vi "Reef Align Play Path Field Position.vi"(1 "PID Constants swerve":T1={"P Gain"=0.09, "I Gain"=0.0, "D Gain"=0.0, "F Gain"=0.08, "I Zone"=0.0, "Min Output"=-1.0, "Max Output"=1.0}, 2 "Operation":T2=enum."Reef Align", 3 "Auto Data":T14={"Auto Velocities"=[{"X Velocity"=-1.8462498434907955, "Y Velocity"=7.056933814139086, "Rotational \nVelocity"=-0.0}, {"X Velocity"=-1.991747061129249, "Y Velocity"=7.535671418858484, "Rotational \nVelocity"=-7.2}, {"X Velocity"=-2.1476402119148625, "Y Velocity"=8.011584634482254, "Rotational \nVelocity"=-10.052643775939941}, {"X Velocity"=-2.306896278662117, "Y Velocity"=8.486490625788083, "Rotational \nVelocity"=-10.052643775939941}, {"X Velocity"=-2.4695100913190724, "Y Velocity"=8.960371657345226, "Rotational \nVelocity"=-10.052643775939941}, {"X Velocity"=-2.635476396794092, "Y Velocity"=9.433210017677535, "Rotational \nVelocity"=-10.052643775939941}, {"X Velocity"=-2.6685615639393947, "Y Velocity"=9.423903981638178, "Rotational \nVelocity"=-10.052643775939941}, {"X Velocity"=-2.701613872254829, "Y Velocity"=9.414481906133277, "Rotational \nVelocity"=-10.052643775939941}, {"X Velocity"=-2.7346329147570203, "Y Velocity"=9.404943907179781, "Rotational \nVelocity"=-10.052643775939941}, {"X Velocity"=-2.6263332099505634, "Y Velocity"=8.91566678376851, "Rotational \nVelocity"=-10.052643775939941}, {"X Velocity"=-2.5146351435076726, "Y Velocity"=8.427271425386172, "Rotational \nVelocity"=-10.052643775939941}, {"X Velocity"=-2.3995435908884546, "Y Velocity"=7.939775651158667, "Rotational \nVelocity"=-10.052643775939941}, {"X Velocity"=-2.2810635107418573, "Y Velocity"=7.453197256780454, "Rotational \nVelocity"=-10.052643775939941}, {"X Velocity"=-2.1591999448009993, "Y Velocity"=6.967554014150215, "Rotational \nVelocity"=-10.052643775939941}, {"X Velocity"=-2.0339580177769934, "Y Velocity"=6.482863671006963, "Rotational \nVelocity"=-10.052643775939941}, {"X Velocity"=-1.9053429372511914, "Y Velocity"=5.99914395056661, "Rotational \nVelocity"=-10.052643775939941}, {"X Velocity"=-1.7733599935659488, "Y Velocity"=5.516412551158996, "Rotational \nVelocity"=-10.052643775939941}, {"X Velocity"=-1.63801455971383, "Y Velocity"=5.034687145865371, "Rotational \nVelocity"=-10.052643775939941}, {"X Velocity"=-1.4993120912253046, "Y Velocity"=4.553985382156366, "Rotational \nVelocity"=-10.052643775939941}, {"X Velocity"=-1.3572581260549188, "Y Velocity"=4.074324881530425, "Rotational \nVelocity"=-10.052643775939941}, {"X Velocity"=-1.2118582844659433, "Y Velocity"=3.595723239152738, "Rotational \nVelocity"=-10.052643775939941}, {"X Velocity"=-1.0631182689134988, "Y Velocity"=3.118198023494648, "Rotational \nVelocity"=-10.052643775939941}, {"X Velocity"=-0.9110438639261721, "Y Velocity"=2.641766775973572, "Rotational \nVelocity"=-10.052643775939941}, {"X Velocity"=-0.7556409359861169, "Y Velocity"=2.166447010593411, "Rotational \nVelocity"=-10.052643775939941}, {"X Velocity"=-0.5969154334076338, "Y Velocity"=1.692256213585474, "Rotational \nVelocity"=-10.052643775939941}, {"X Velocity"=-0.4348733862142511, "Y Velocity"=1.2192118430499221, "Rotational \nVelocity"=-10.052643775939941}, {"X Velocity"=-0.26947258503234844, "Y Velocity"=0.7473487535270189, "Rotational \nVelocity"=-9.867414283752396}, {"X Velocity"=-0.1001328097589842, "Y Velocity"=0.2768976473427397, "Rotational \nVelocity"=-2.6674142837523886}, {"X Velocity"=-0.0, "Y Velocity"=0.0, "Rotational \nVelocity"=-0.0}], "Auto Positions"=[{"x"=0.8100058273974486, "y"=-3.967975741983552, "th"=5.222202301025391}, {"x"=0.7603878706355013, "y"=-3.830783760791278, "th"=5.0782023010253905}, {"x"=0.7073688364180365, "y"=-3.68418791485404, "th"=4.877149425506592}, {"x"=0.6509487247450543, "y"=-3.5281882041718386, "th"=4.676096549987793}, {"x"=0.5911275356165546, "y"=-3.3627846287446737, "th"=4.475043674468994}, {"x"=0.5279052690325376, "y"=-3.1879771885725448, "th"=4.273990798950195}, {"x"=0.46128192499300325, "y"=-3.0037658836554524, "th"=4.072937923431397}, {"x"=0.39465858095346884, "y"=-2.8195545787383596, "th"=3.8718850479125977}, {"x"=0.32803523691393444, "y"=-2.6353432738212668, "th"=3.6708321723937987}, {"x"=0.26141189287440003, "y"=-2.451131968904174, "th"=3.469779296875}, {"x"=0.198189626290383, "y"=-2.276324528732045, "th"=3.2687264213562015}, {"x"=0.1383684371618834, "y"=-2.1109209533048796, "th"=3.0676735458374025}, {"x"=0.0819483254889012, "y"=-1.954921242622678, "th"=2.8666206703186035}, {"x"=0.02892929127143639, "y"=-1.8083253966854402, "th"=2.6655677947998044}, {"x"=-0.020688665490511016, "y"=-1.671133415493166, "th"=2.4645149192810054}, {"x"=-0.06690554479694102, "y"=-1.5433452990458556, "th"=2.2634620437622064}, {"x"=-0.10972134664785363, "y"=-1.4249610473435088, "th"=2.0624091682434074}, {"x"=-0.14913607104324883, "y"=-1.315980660386126, "th"=1.8613562927246083}, {"x"=-0.18514971798312663, "y"=-1.2164041381737067, "th"=1.6603034172058093}, {"x"=-0.21776228746748705, "y"=-1.1262314807062512, "th"=1.4592505416870103}, {"x"=-0.24697377949633004, "y"=-1.0454626879837594, "th"=1.2581976661682113}, {"x"=-0.27278419406965565, "y"=-0.9740977600062313, "th"=1.0571447906494127}, {"x"=-0.29519353118746383, "y"=-0.9121366967736668, "th"=0.8560919151306141}, {"x"=-0.31420179084975464, "y"=-0.8595794982860661, "th"=0.6550390396118155}, {"x"=-0.329808973056528, "y"=-0.816426164543429, "th"=0.45398616409301695}, {"x"=-0.342015077807784, "y"=-0.7826766955457557, "th"=0.2529332885742184}, {"x"=-0.35082010510352263, "y"=-0.7583310912930461, "th"=0.055585002899170455}, {"x"=-0.3562240549437438, "y"=-0.7433893517853002, "th"=0.002236717224122664}, {"x"=-0.35822692732844763, "y"=-0.737851477022518, "th"=0.002236717224122664}], "Auto Commands"=[], "Zero Velocity?"=[]}, 4 "Motors":T3={"Drive Motors (NEO)"={"Left Front"={"DeviceStatus"={"status"=FALSE, "code"=0, "source"=""}, "Type"=enum."CAN", "PWM"={"PWM Channel"=enum."Invalid", "DeadBand"={"Name"="", "maxPositivePwm"=0, "minPositivePwm"=0, "centerPwm"=0, "maxNegativePwm"=0, "minNegativePwm"=0, "angularRange"=0}}, "CAN"={"Device Number"=1, "SetOutput VI Ref"=variant(refnum<vi> refnum), "GetOutput VI Ref"=variant(refnum<vi> refnum), "Enable VI Ref"=variant(refnum<vi> refnum), "Disable VI Ref"=variant(refnum<vi> refnum), "Data"=variant(cluster{"Ext ID":u32, "CAN Timeout":u32, "Inverted No WPILib":bool, "Has Configured Limit Sw":bool, "Has Configured Alt Encoder":bool, "SPARK Model":enum16{"SPARK MAX", "SPARK Flex", "Unknown"}, "CAN Max Retries":u32, "CAN Timeout (ms)":u32, "Status 0 Period (ms)":u32, "Status 1 Period (ms)":u32, "Status 2 Period (ms)":u32, "Status 3 Period (ms)":u32, "Status 4 Period (ms)":u32, "Status 5 Period (ms)":u32, "Status 6 Period (ms)":u32, "Status 7 Period (ms)":u32, "Status Frame Timeout (ms)":u32} {"Ext ID"=33882113, "CAN Timeout"=0, "Inverted No WPILib"=FALSE, "Has Configured Limit Sw"=FALSE, "Has Configured Alt Encoder"=FALSE, "SPARK Model"=enum."SPARK Flex", "CAN Max Retries"=5, "CAN Timeout (ms)"=20, "Status 0 Period (ms)"=10, "Status 1 Period (ms)"=250, "Status 2 Period (ms)"=20, "Status 3 Period (ms)"=20, "Status 4 Period (ms)"=20, "Status 5 Period (ms)"=20, "Status 6 Period (ms)"=20, "Status 7 Period (ms)"=20, "Status Frame Timeout (ms)"=500})}, "Invert"=FALSE, "DIO PWM"={"PWM \"Enable\" Channel"=enum."Invalid", "DIOChannel"=enum."Invalid", "PWM Rate"=0.0}}, "Left Back"={"DeviceStatus"={"status"=FALSE, "code"=0, "source"=""}, "Type"=enum."CAN", "PWM"={"PWM Channel"=enum."Invalid", "DeadBand"={"Name"="", "maxPositivePwm"=0, "minPositivePwm"=0, "centerPwm"=0, "maxNegativePwm"=0, "minNegativePwm"=0, "angularRange"=0}}, "CAN"={"Device Number"=3, "SetOutput VI Ref"=variant(refnum<vi> refnum), "GetOutput VI Ref"=variant(refnum<vi> refnum), "Enable VI Ref"=variant(refnum<vi> refnum), "Disable VI Ref"=variant(refnum<vi> refnum), "Data"=variant(cluster{"Ext ID":u32, "CAN Timeout":u32, "Inverted No WPILib":bool, "Has Configured Limit Sw":bool, "Has Configured Alt Encoder":bool, "SPARK Model":enum16{"SPARK MAX", "SPARK Flex", "Unknown"}, "CAN Max Retries":u32, "CAN Timeout (ms)":u32, "Status 0 Period (ms)":u32, "Status 1 Period (ms)":u32, "Status 2 Period (ms)":u32, "Status 3 Period (ms)":u32, "Status 4 Period (ms)":u32, "Status 5 Period (ms)":u32, "Status 6 Period (ms)":u32, "Status 7 Period (ms)":u32, "Status Frame Timeout (ms)":u32} {"Ext ID"=33882115, "CAN Timeout"=0, "Inverted No WPILib"=FALSE, "Has Configured Limit Sw"=FALSE, "Has Configured Alt Encoder"=FALSE, "SPARK Model"=enum."SPARK Flex", "CAN Max Retries"=5, "CAN Timeout (ms)"=20, "Status 0 Period (ms)"=10, "Status 1 Period (ms)"=250, "Status 2 Period (ms)"=20, "Status 3 Period (ms)"=20, "Status 4 Period (ms)"=20, "Status 5 Period (ms)"=20, "Status 6 Period (ms)"=20, "Status 7 Period (ms)"=20, "Status Frame Timeout (ms)"=500})}, "Invert"=FALSE, "DIO PWM"={"PWM \"Enable\" Channel"=enum."Invalid", "DIOChannel"=enum."Invalid", "PWM Rate"=0.0}}, "Right Front"={"DeviceStatus"={"status"=FALSE, "code"=0, "source"=""}, "Type"=enum."CAN", "PWM"={"PWM Channel"=enum."Invalid", "DeadBand"={"Name"="", "maxPositivePwm"=0, "minPositivePwm"=0, "centerPwm"=0, "maxNegativePwm"=0, "minNegativePwm"=0, "angularRange"=0}}, "CAN"={"Device Number"=5, "SetOutput VI Ref"=variant(refnum<vi> refnum), "GetOutput VI Ref"=variant(refnum<vi> refnum), "Enable VI Ref"=variant(refnum<vi> refnum), "Disable VI Ref"=variant(refnum<vi> refnum), "Data"=variant(cluster{"Ext ID":u32, "CAN Timeout":u32, "Inverted No WPILib":bool, "Has Configured Limit Sw":bool, "Has Configured Alt Encoder":bool, "SPARK Model":enum16{"SPARK MAX", "SPARK Flex", "Unknown"}, "CAN Max Retries":u32, "CAN Timeout (ms)":u32, "Status 0 Period (ms)":u32, "Status 1 Period (ms)":u32, "Status 2 Period (ms)":u32, "Status 3 Period (ms)":u32, "Status 4 Period (ms)":u32, "Status 5 Period (ms)":u32, "Status 6 Period (ms)":u32, "Status 7 Period (ms)":u32, "Status Frame Timeout (ms)":u32} {"Ext ID"=33882117, "CAN Timeout"=0, "Inverted No WPILib"=FALSE, "Has Configured Limit Sw"=FALSE, "Has Configured Alt Encoder"=FALSE, "SPARK Model"=enum."SPARK Flex", "CAN Max Retries"=5, "CAN Timeout (ms)"=20, "Status 0 Period (ms)"=10, "Status 1 Period (ms)"=250, "Status 2 Period (ms)"=20, "Status 3 Period (ms)"=20, "Status 4 Period (ms)"=20, "Status 5 Period (ms)"=20, "Status 6 Period (ms)"=20, "Status 7 Period (ms)"=20, "Status Frame Timeout (ms)"=500})}, "Invert"=FALSE, "DIO PWM"={"PWM \"Enable\" Channel"=enum."Invalid", "DIOChannel"=enum."Invalid", "PWM Rate"=0.0}}, "Right Back"={"DeviceStatus"={"status"=FALSE, "code"=0, "source"=""}, "Type"=enum."CAN", "PWM"={"PWM Channel"=enum."Invalid", "DeadBand"={"Name"="", "maxPositivePwm"=0, "minPositivePwm"=0, "centerPwm"=0, "maxNegativePwm"=0, "minNegativePwm"=0, "angularRange"=0}}, "CAN"={"Device Number"=7, "SetOutput VI Ref"=variant(refnum<vi> refnum), "GetOutput VI Ref"=variant(refnum<vi> refnum), "Enable VI Ref"=variant(refnum<vi> refnum), "Disable VI Ref"=variant(refnum<vi> refnum), "Data"=variant(cluster{"Ext ID":u32, "CAN Timeout":u32, "Inverted No WPILib":bool, "Has Configured Limit Sw":bool, "Has Configured Alt Encoder":bool, "SPARK Model":enum16{"SPARK MAX", "SPARK Flex", "Unknown"}, "CAN Max Retries":u32, "CAN Timeout (ms)":u32, "Status 0 Period (ms)":u32, "Status 1 Period (ms)":u32, "Status 2 Period (ms)":u32, "Status 3 Period (ms)":u32, "Status 4 Period (ms)":u32, "Status 5 Period (ms)":u32, "Status 6 Period (ms)":u32, "Status 7 Period (ms)":u32, "Status Frame Timeout (ms)":u32} {"Ext ID"=33882119, "CAN Timeout"=0, "Inverted No WPILib"=FALSE, "Has Configured Limit Sw"=FALSE, "Has Configured Alt Encoder"=FALSE, "SPARK Model"=enum."SPARK Flex", "CAN Max Retries"=5, "CAN Timeout (ms)"=20, "Status 0 Period (ms)"=10, "Status 1 Period (ms)"=250, "Status 2 Period (ms)"=20, "Status 3 Period (ms)"=20, "Status 4 Period (ms)"=20, "Status 5 Period (ms)"=20, "Status 6 Period (ms)"=20, "Status 7 Period (ms)"=20, "Status Frame Timeout (ms)"=500})}, "Invert"=FALSE, "DIO PWM"={"PWM \"Enable\" Channel"=enum."Invalid", "DIOChannel"=enum."Invalid", "PWM Rate"=0.0}}}, "Steer Motors (NEO)"={"Left Front"={"DeviceStatus"={"status"=FALSE, "code"=0, "source"=""}, "Type"=enum."CAN", "PWM"={"PWM Channel"=enum."Invalid", "DeadBand"={"Name"="", "maxPositivePwm"=0, "minPositivePwm"=0, "centerPwm"=0, "maxNegativePwm"=0, "minNegativePwm"=0, "angularRange"=0}}, "CAN"={"Device Number"=2, "SetOutput VI Ref"=variant(refnum<vi> refnum), "GetOutput VI Ref"=variant(refnum<vi> refnum), "Enable VI Ref"=variant(refnum<vi> refnum), "Disable VI Ref"=variant(refnum<vi> refnum), "Data"=variant(cluster{"Ext ID":u32, "CAN Timeout":u32, "Inverted No WPILib":bool, "Has Configured Limit Sw":bool, "Has Configured Alt Encoder":bool, "SPARK Model":enum16{"SPARK MAX", "SPARK Flex", "Unknown"}, "CAN Max Retries":u32, "CAN Timeout (ms)":u32, "Status 0 Period (ms)":u32, "Status 1 Period (ms)":u32, "Status 2 Period (ms)":u32, "Status 3 Period (ms)":u32, "Status 4 Period (ms)":u32, "Status 5 Period (ms)":u32, "Status 6 Period (ms)":u32, "Status 7 Period (ms)":u32, "Status Frame Timeout (ms)":u32} {"Ext ID"=33882114, "CAN Timeout"=0, "Inverted No WPILib"=TRUE, "Has Configured Limit Sw"=FALSE, "Has Configured Alt Encoder"=FALSE, "SPARK Model"=enum."SPARK MAX", "CAN Max Retries"=5, "CAN Timeout (ms)"=20, "Status 0 Period (ms)"=10, "Status 1 Period (ms)"=250, "Status 2 Period (ms)"=20, "Status 3 Period (ms)"=20, "Status 4 Period (ms)"=20, "Status 5 Period (ms)"=20, "Status 6 Period (ms)"=20, "Status 7 Period (ms)"=20, "Status Frame Timeout (ms)"=500})}, "Invert"=FALSE, "DIO PWM"={"PWM \"Enable\" Channel"=enum."Invalid", "DIOChannel"=enum."Invalid", "PWM Rate"=0.0}}, "Left Back"={"DeviceStatus"={"status"=FALSE, "code"=0, "source"=""}, "Type"=enum."CAN", "PWM"={"PWM Channel"=enum."Invalid", "DeadBand"={"Name"="", "maxPositivePwm"=0, "minPositivePwm"=0, "centerPwm"=0, "maxNegativePwm"=0, "minNegativePwm"=0, "angularRange"=0}}, "CAN"={"Device Number"=4, "SetOutput VI Ref"=variant(refnum<vi> refnum), "GetOutput VI Ref"=variant(refnum<vi> refnum), "Enable VI Ref"=variant(refnum<vi> refnum), "Disable VI Ref"=variant(refnum<vi> refnum), "Data"=variant(cluster{"Ext ID":u32, "CAN Timeout":u32, "Inverted No WPILib":bool, "Has Configured Limit Sw":bool, "Has Configured Alt Encoder":bool, "SPARK Model":enum16{"SPARK MAX", "SPARK Flex", "Unknown"}, "CAN Max Retries":u32, "CAN Timeout (ms)":u32, "Status 0 Period (ms)":u32, "Status 1 Period (ms)":u32, "Status 2 Period (ms)":u32, "Status 3 Period (ms)":u32, "Status 4 Period (ms)":u32, "Status 5 Period (ms)":u32, "Status 6 Period (ms)":u32, "Status 7 Period (ms)":u32, "Status Frame Timeout (ms)":u32} {"Ext ID"=33882116, "CAN Timeout"=0, "Inverted No WPILib"=TRUE, "Has Configured Limit Sw"=FALSE, "Has Configured Alt Encoder"=FALSE, "SPARK Model"=enum."SPARK MAX", "CAN Max Retries"=5, "CAN Timeout (ms)"=20, "Status 0 Period (ms)"=10, "Status 1 Period (ms)"=250, "Status 2 Period (ms)"=20, "Status 3 Period (ms)"=20, "Status 4 Period (ms)"=20, "Status 5 Period (ms)"=20, "Status 6 Period (ms)"=20, "Status 7 Period (ms)"=20, "Status Frame Timeout (ms)"=500})}, "Invert"=FALSE, "DIO PWM"={"PWM \"Enable\" Channel"=enum."Invalid", "DIOChannel"=enum."Invalid", "PWM Rate"=0.0}}, "Right Front"={"DeviceStatus"={"status"=FALSE, "code"=0, "source"=""}, "Type"=enum."CAN", "PWM"={"PWM Channel"=enum."Invalid", "DeadBand"={"Name"="", "maxPositivePwm"=0, "minPositivePwm"=0, "centerPwm"=0, "maxNegativePwm"=0, "minNegativePwm"=0, "angularRange"=0}}, "CAN"={"Device Number"=6, "SetOutput VI Ref"=variant(refnum<vi> refnum), "GetOutput VI Ref"=variant(refnum<vi> refnum), "Enable VI Ref"=variant(refnum<vi> refnum), "Disable VI Ref"=variant(refnum<vi> refnum), "Data"=variant(cluster{"Ext ID":u32, "CAN Timeout":u32, "Inverted No WPILib":bool, "Has Configured Limit Sw":bool, "Has Configured Alt Encoder":bool, "SPARK Model":enum16{"SPARK MAX", "SPARK Flex", "Unknown"}, "CAN Max Retries":u32, "CAN Timeout (ms)":u32, "Status 0 Period (ms)":u32, "Status 1 Period (ms)":u32, "Status 2 Period (ms)":u32, "Status 3 Period (ms)":u32, "Status 4 Period (ms)":u32, "Status 5 Period (ms)":u32, "Status 6 Period (ms)":u32, "Status 7 Period (ms)":u32, "Status Frame Timeout (ms)":u32} {"Ext ID"=33882118, "CAN Timeout"=0, "Inverted No WPILib"=TRUE, "Has Configured Limit Sw"=FALSE, "Has Configured Alt Encoder"=FALSE, "SPARK Model"=enum."SPARK MAX", "CAN Max Retries"=5, "CAN Timeout (ms)"=20, "Status 0 Period (ms)"=10, "Status 1 Period (ms)"=250, "Status 2 Period (ms)"=20, "Status 3 Period (ms)"=20, "Status 4 Period (ms)"=20, "Status 5 Period (ms)"=20, "Status 6 Period (ms)"=20, "Status 7 Period (ms)"=20, "Status Frame Timeout (ms)"=500})}, "Invert"=FALSE, "DIO PWM"={"PWM \"Enable\" Channel"=enum."Invalid", "DIOChannel"=enum."Invalid", "PWM Rate"=0.0}}, "Right Back"={"DeviceStatus"={"status"=FALSE, "code"=0, "source"=""}, "Type"=enum."CAN", "PWM"={"PWM Channel"=enum."Invalid", "DeadBand"={"Name"="", "maxPositivePwm"=0, "minPositivePwm"=0, "centerPwm"=0, "maxNegativePwm"=0, "minNegativePwm"=0, "angularRange"=0}}, "CAN"={"Device Number"=8, "SetOutput VI Ref"=variant(refnum<vi> refnum), "GetOutput VI Ref"=variant(refnum<vi> refnum), "Enable VI Ref"=variant(refnum<vi> refnum), "Disable VI Ref"=variant(refnum<vi> refnum), "Data"=variant(cluster{"Ext ID":u32, "CAN Timeout":u32, "Inverted No WPILib":bool, "Has Configured Limit Sw":bool, "Has Configured Alt Encoder":bool, "SPARK Model":enum16{"SPARK MAX", "SPARK Flex", "Unknown"}, "CAN Max Retries":u32, "CAN Timeout (ms)":u32, "Status 0 Period (ms)":u32, "Status 1 Period (ms)":u32, "Status 2 Period (ms)":u32, "Status 3 Period (ms)":u32, "Status 4 Period (ms)":u32, "Status 5 Period (ms)":u32, "Status 6 Period (ms)":u32, "Status 7 Period (ms)":u32, "Status Frame Timeout (ms)":u32} {"Ext ID"=33882120, "CAN Timeout"=0, "Inverted No WPILib"=TRUE, "Has Configured Limit Sw"=FALSE, "Has Configured Alt Encoder"=FALSE, "SPARK Model"=enum."SPARK MAX", "CAN Max Retries"=5, "CAN Timeout (ms)"=20, "Status 0 Period (ms)"=10, "Status 1 Period (ms)"=250, "Status 2 Period (ms)"=20, "Status 3 Period (ms)"=20, "Status 4 Period (ms)"=20, "Status 5 Period (ms)"=20, "Status 6 Period (ms)"=20, "Status 7 Period (ms)"=20, "Status Frame Timeout (ms)"=500})}, "Invert"=FALSE, "DIO PWM"={"PWM \"Enable\" Channel"=enum."Invalid", "DIOChannel"=enum."Invalid", "PWM Rate"=0.0}}}, "Pigeon2"={"DeviceStatus"={"status"=FALSE, "code"=0, "source"=""}, "Device Number"=21, "Type"=352321536, "Device ID"=352321557, "Handle"=22044056, "UsageFrame"=0, "Library Path"=path "libCTRE_PhoenixCCI.so"}, "Radii (ft)"={"Left Front Position"=[-0.9375, 0.9375], "Left Back Position"=[-0.9375, -0.9375], "Right Front Position"=[0.9375, 0.9375], "Right Back Position"=[0.9375, -0.9375]}} {"Radii (ft)"."Right Back Position" format="%.2f"; "Radii (ft)"."Right Front Position" format="%.2f"; "Radii (ft)"."Left Back Position" format="%.2f"; "Radii (ft)"."Left Front Position" format="%.2f"; "Pigeon2"."Type" items=["CAN"=352321536, "TalonSRX"=33554432]}) -> (0 "Align Good?":bool)   [LabVIEW 2023]
uses:
  swerve/Type Definitions/Data/Robot Velocities.ctl
  swerve/Type Definitions/Hardware/Swerve Drives/(NEO-NEO-ThroughBore-Pigeon2) Swerve.ctl
  swerve/Type Definitions/Hardware/4 Motor Sets/(NEO & NEO 550) 4 Motor Set.ctl
  <vilib>/Rock Robotics/WPI/MotorControl/WPI_MotorControlDeviceRef.ctl
  <vilib>/Rock Robotics/WPI/MotorControl/WPI_MotorControlType.ctl
  <vilib>/Rock Robotics/SystemInterfaces/DIO/FPGA_DIOPWMChannel.ctl
  <vilib>/Rock Robotics/WPI/PWM/WPI_PWMDeadband.ctl
  <vilib>/Rock Robotics/SystemInterfaces/DIO/FPGA_DIOChannel.ctl
  <vilib>/Rock Robotics/WPI/ThirdParty/Phoenix-LabVIEW/Pigeon IMU/CTRE_PigeonIMU_DeviceRef.ctl
  <vilib>/Rock Robotics/WPI/ThirdParty/Phoenix-LabVIEW/Pigeon IMU/CTRE_PigeonIMU_ConnectionType.ctl
  swerve/Type Definitions/Data/Pod Positions.ctl
  Implementation/Drive Operations.ctl
  <vilib>/Rock Robotics/WPI/ThirdParty/REV Robotics/REVLib/Typedef/Spark MAX Control Type.ctl
  <vilib>/Platform/TimedLoop/XDataNode/timing_clust.ctl
  <vilib>/Platform/TimedLoop/XDataNode/nitl_modes.ctl
  <vilib>/Platform/TimedLoop/XDataNode/wakeup.ctl
  <vilib>/Rock Robotics/WPI/DriverStation/WPI_DriverStationRobotMode2.ctl
  ba9e1e52-2e86-4a5f-ad71-bc975f8651a0.vi
  Framework/Robot Global Data.vi
  <vilib>/Platform/TimedLoop/XDataNode/XDataNode.xnode
  <vilib>/Platform/TimedLoop/XDataNode/XDNodeRunTimeDep.lvlib
panel:
  out "Delay":dbl=9.0
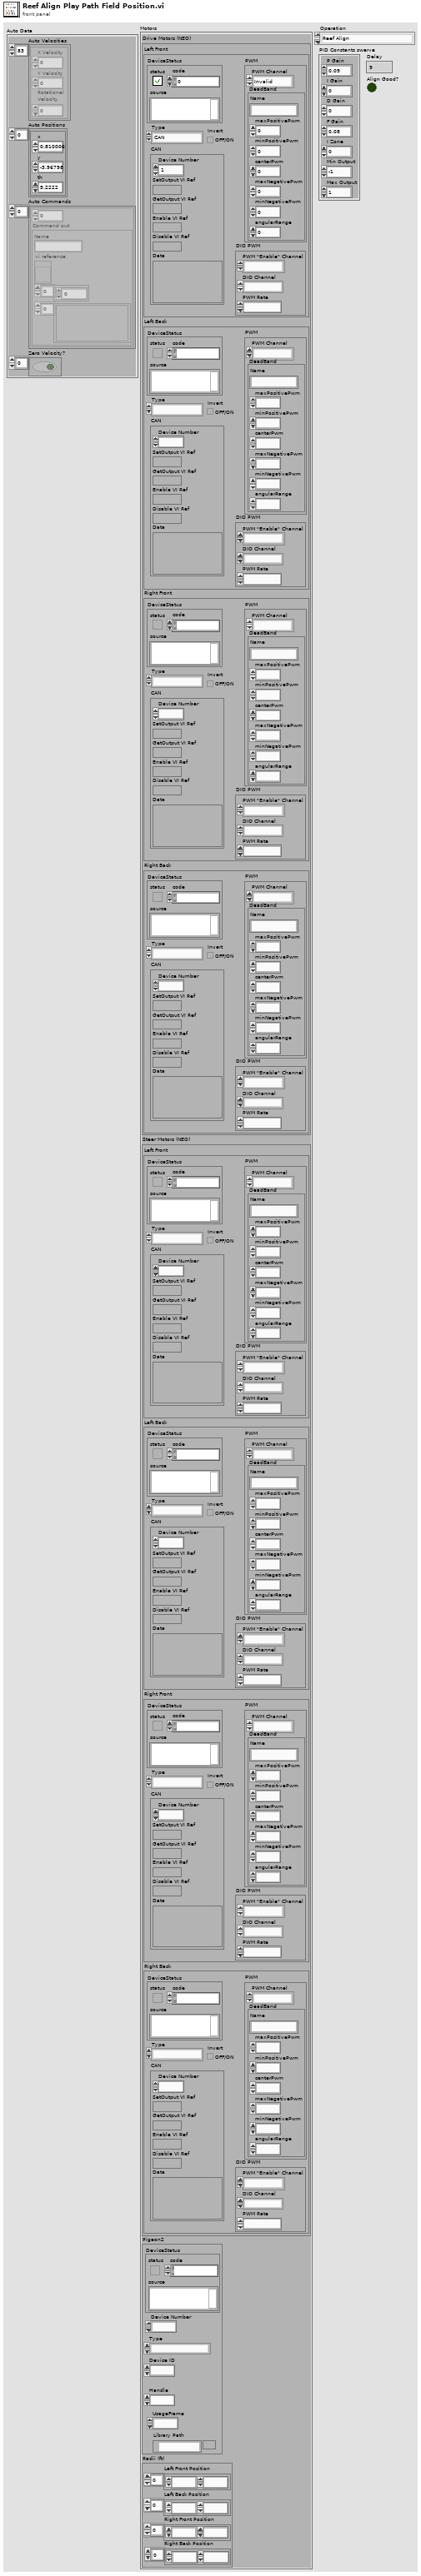
[diagram p1: front panel]
types:
  T1 = cluster{"P Gain":dbl, "I Gain":dbl, "D Gain":dbl, "F Gain":dbl, "I Zone":dbl, "Min Output":dbl, "Max Output":dbl}
  T2 = typedef "Drive Operations.ctl" = enum16{"Reserve", "Read Current", "Immediate", "Calibrate", "Reef Align", "Auto", "Old Reef Align"}
  T3 = typedef "(NEO-NEO-ThroughBore-Pigeon2) Swerve.ctl" = cluster{"Drive Motors (NEO)":T4, "Steer Motors (NEO)":T4, "Pigeon2":T10, "Radii (ft)":T12}
  T4 = typedef "(NEO & NEO 550) 4 Motor Set.ctl" = cluster{"Left Front":T5, "Left Back":T5, "Right Front":T5, "Right Back":T5}
  T5 = typedef "WPI_MotorControlDeviceRef.ctl" = cluster{"DeviceStatus":errorcluster, "Type":T6, "PWM":cluster{"PWM Channel":T7, "DeadBand":T8}, "CAN":cluster{"Device Number":u8, "SetOutput VI Ref":variant, "GetOutput VI Ref":variant, "Enable VI Ref":variant, "Disable VI Ref":variant, "Data":variant}, "Invert":bool, "DIO PWM":cluster{"PWM \"Enable\" Channel":T7, "DIOChannel":T9, "PWM Rate":dbl}}
  T6 = typedef "WPI_MotorControlType.ctl" = enum16{"PWM", "CAN", "DIO PWM"}
  T7 = typedef "FPGA_DIOPWMChannel.ctl" = enum8{"PWM 0", "PWM 1", "PWM 2", "PWM 3", "PWM 4", "PWM 5", "PWM 6", "PWM 7", "PWM 8", "PWM 9", "PWM MXP 0", "PWM MXP 1", "PWM MXP 2", "PWM MXP 3", "PWM MXP 4", "PWM MXP 5", "PWM MXP 6", "PWM MXP 7", "PWM MXP 8", "PWM MXP 9", "Invalid"}
  T8 = typedef "WPI_PWMDeadband.ctl" = cluster{"Name":string, "maxPositivePwm":i32, "minPositivePwm":i32, "centerPwm":i32, "maxNegativePwm":i32, "minNegativePwm":i32, "angularRange":u16}
  T9 = typedef "FPGA_DIOChannel.ctl" = enum8{"DIO 0", "DIO 1", "DIO 2", "DIO 3", "DIO 4", "DIO 5", "DIO 6", "DIO 7", "DIO 8", "DIO 9", "DIO MXP 0", "DIO MXP 1", "DIO MXP 2", "DIO MXP 3", "DIO MXP 4", "DIO MXP 5", "DIO MXP 6", "DIO MXP 7", "DIO MXP 8", "DIO MXP 9", "DIO MXP 10", "DIO MXP 11", "DIO MXP 12", "DIO MXP 13", "DIO MXP 14", "DIO MXP 15", "SPI Port CS1", "SPI Port CS2", "SPI Port CS3", "SPI Port MISO", "SPI Port MOSI", "Invalid"}
  T10 = typedef "CTRE_PigeonIMU_DeviceRef.ctl" = cluster{"DeviceStatus":errorcluster, "Device Number":u8, "Type":T11, "Device ID":u32, "Handle":u64, "UsageFrame":u32, "Library Path":path}
  T11 = typedef "CTRE_PigeonIMU_ConnectionType.ctl" = u32
  T12 = typedef "Pod Positions.ctl" = cluster{"Left Front Position":dbl[], "Left Back Position":dbl[], "Right Front Position":dbl[], "Right Back Position":dbl[]}
  T13 = typedef "Robot Velocities.ctl" = cluster{"X Velocity":dbl, "Y Velocity":dbl, "Rotational \nVelocity":dbl}
  T14 = cluster{"Auto Velocities":T13[], "Auto Positions":cluster{"x":dbl, "y":dbl, "th":dbl}[], "Auto Commands":cluster{dbl, "Command out":cluster{"Name":string, "vi reference":refnum<vi>, i32[], variant[]}}[], "Zero Velocity?":bool[]}
  T15 = typedef "Spark MAX Control Type.ctl" = enum16{"Percent VBus", "Voltage", "Velocity", "Position", "Smart Motion", "Current", "Smart Velocity", "MAXMotion Position", "MAXMotion Velocity"}
  T16 = cluster{"Left Front":dbl, "Left Back":dbl, "Right Front":dbl, "Right Back":dbl}
  T17 = cluster{"Time (s)":dbl, "Command out":cluster{"Name":string, "vi reference":refnum<vi>, i32[], variant[]}}
  T18 = cluster{dbl, "Command out":cluster{"Name":string, "vi reference":refnum<vi>, i32[], variant[]}}[]
  T19 = typedef "XDNodeRunTimeDep.lvlib/timing_clust.ctl" = cluster{"Expected End [f-1]":u64, "Actual End [f-1]":u64, "Finished Late? [f-1]":bool, "Expected End [i-1]":u64, "Actual End [i-1]":u64, "Finished Late? [i-1]":bool, "Expected Start [i]":u64, "Actual Start [i]":u64, "Expected Start [f]":u64, "Actual Start [f]":u64, "Source Name":string, "Structure Name":string, "Period":i64, "Deadline":i64, "Offset":i64, "Start":i64, "Priority":i32, "Timeout":i32, "Mode":T20, "Wakeup Reason":T21, "Error":errorcluster, "Source Type":string, "Secondary Source Type":string, "Global End Time":u64, "Global Start Time":u64, "Frame Duration":u64, "Iteration Duration":u64, "Assigned CPU":i32, "I/O Scan Engine Mode":u32}
  T20 = typedef "XDNodeRunTimeDep.lvlib/nitl_modes.ctl" = enum32{"No Change", "Process missed periods, maintain original phase", "Discard missed periods, maintain original phase", "Process missed periods, ignore original phase", "Discard missed periods, ignore original phase"}
  T21 = typedef "XDNodeRunTimeDep.lvlib/wakeup.ctl" = enum32{"Normal", "Aborted", "Asynchronous wakeup", "Timing source error", "Timed loop error", "Timeout"}
  T22 = cluster{"Field Centric":bool, "Reef Centric":bool}
  T23 = typedef "WPI_DriverStationRobotMode2.ctl" = enum16{"Autonomous Disabled", "Autonomous Enabled", "Teleop Disabled", "Teleop Enabled", "Disconnected", "Finish", "Test Disabled", "Test Enabled", "Emergency Stopped"}
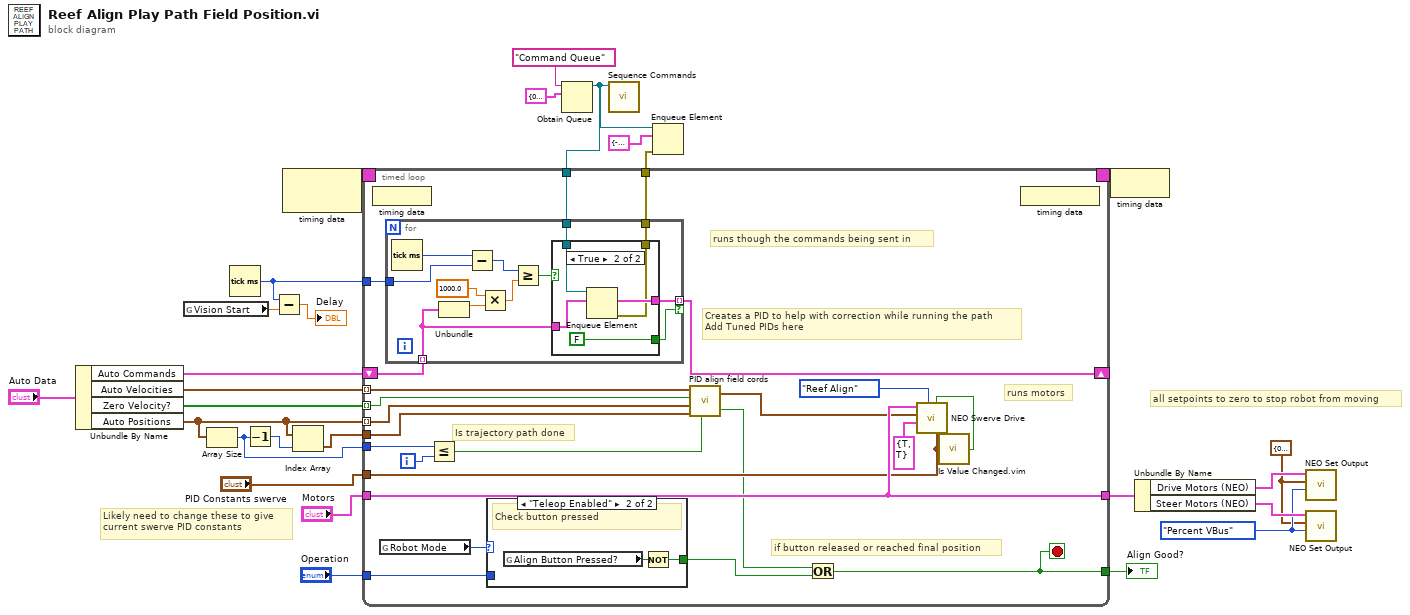
[diagram p0: block diagram]
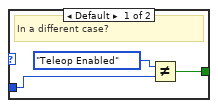
[diagram p2: hidden frame]
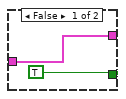
[diagram p3: hidden frame]
diagram:
  w12 = Spark_MAX_Control_Type."Percent VBus" ("Control Mode")
  w11 = T16 {"Left Front"=0.0, "Left Back"=0.0, "Right Front"=0.0, "Right Back"=0.0} ("Setpoints")
  # "Likely need to change these to give \ncurrent swerve PID constants"
  # "all setpoints to zero to stop robot from moving"
  n1 = Unbundle By Name("Auto Data") -> ("Auto Commands"=w16:T18, "Auto Velocities"=w7:T13[], "Zero Velocity?"=w15:bool[], "Auto Positions"=w6:cluster{"x":dbl, "y":dbl, "th":dbl}[])
  n2 = global read "Robot Global Data.vi" "Vision Start"() -> (w27:dbl)
  n3 = Array Size(array=w6) -> (size(s)=w4:i32)
  n4 = Tick Count (ms)() -> (millisecond timer value=w18:u32)
  n5 = Decrement(x=w4) -> (x-1=w5:i32)
  n6 = Subtract(x=w18, y=w27) -> (x-y=→"Delay":dbl)
  n7 = node-c288() -> (w25:T19)  [unwired: 1 in]
  n8 = Index Array(array=w6, index=w5) -> (element=w1:cluster{"x":dbl, "y":dbl, "th":dbl})
  n9 = Obtain Queue(name (unnamed)="Command Queue", element data type=T17 {"Time (s)"=0.0, "Command out"={"Name"="", "vi reference"=refnum, [], []}} ("element")) -> (queue out=w20:refnum<queue>)  [unwired: 3 in, 2 out]
  n10 = timed-loop {
    timing: w25 -> [_]
    timing-out: [_] -> w24
    tunnel: w20 -> [w50]
    tunnel: [w49] -> w19
    tunnel: w18 -> [w47]
    shift-right: [w46] -> _
    shift-left: w16 -> [w48]
    tunnel: w15 -> [w37] mode=indexing
    tunnel: w7 -> [w45] mode=indexing
    tunnel: w6 -> [w38] mode=indexing
    tunnel: "Motors" -> [w42]
    tunnel: [w42] -> w9
    tunnel: "PID Constants swerve" -> [w40]
    tunnel: w1 -> [w36]
    tunnel: w4 -> [w35]
    tunnel: "Operation" -> [w32]
    tunnel: [w31] -> w2
    i -> [w39]
    stop <- w31 stop-if-true
    # "if button released or reached final position"
    # "Is trajectory path done"
    # "runs motors"
    # "Creates a PID to help with correction while running the path\nAdd Tuned PIDs here"
    # "runs though the commands being sent in"
    n11 = node-c288() -> ()  [unwired: 1 in]
    n12 = global read "Robot Global Data.vi" "Robot Mode"() -> (w33:T23)
    n13 = for {
      tunnel: w50 -> [w67]
      tunnel: [w66] -> w46 mode=indexing if=w65
      tunnel: [w64] -> w49
      tunnel: w48 -> [w63] mode=indexing
      tunnel: w47 -> [w57]
      n14 = Tick Count (ms)() -> (millisecond timer value=w59:u32)
      n15 = Unbundle(w63) -> (w62:dbl)  [unwired: 1 out]
      n16 = Subtract(x=w59, y=w57) -> (x-y=w58:u32)
      n17 = Multiply(x=1000.0 ("y"), y=w62) -> (x*y=w60:dbl)
      n18 = Greater Or Equal?(x=w58, y=w60) -> (x >= y?=w56:bool)
      n19 = case shown="True" w56 {
        tunnel: w67 -> [_ w73]
        tunnel: w63 -> [w68 w72]
        tunnel: [w68 w72] -> w66
        tunnel: [TRUE FALSE] -> w65
        tunnel: [_ w70] -> w64
        frame False {
        }
        frame True {
          n20 = Enqueue Element(queue=w73, element=w72) -> (error out=w70:errorcluster)  [unwired: 2 in, 2 out]
        }
      }
    }
    n21 = Less Or Equal?(x=w35, y=w39) -> (x <= y?=w34:bool)
    n22 = case shown="\"Teleop Enabled\"" w33 {
      tunnel: [w53 w54] -> w30
      tunnel: w32 -> [w52 _]
      frame Default {
        # "In a different case?"
        n23 = Not Equal?(x=WPI_DriverStationRobotMode2."Teleop Enabled" ("y"), y=w52) -> (x != y?=w53:bool)
      }
      frame "Teleop Enabled" {
        # "Check button pressed"
        n24 = global read "Robot Global Data.vi" "Align Button Pressed?"() -> (w55:bool)
        n25 = Not(x=w55) -> (.not. x?=w54:bool)
      }
    }
    n26 = call "PID align field cords.vi"("Robot Velocities"=w45, "Zero V"=w37, "Expected Position"=w38, "Final Position"=w36, "Path Finished?"=w34) -> ("Final velocity"=w28:T13, "PID happy"=w29:bool)
    n27 = Or(x=w29, y=w30) -> (x .or. y?=w31:bool)
    n28 = call "Is Value Changed.vim"("value"=w40) -> ("changed or first call?"=w41:bool)
    n29 = call "NEO Swerve Drive.vi"("PID Constants"=w40, "Configure?"=w41, "Operation"=Drive_Operations."Reef Align", "Drive Conditions"=T22 {"Field Centric"=TRUE, "Reef Centric"=TRUE}, "Robot Velocities"=w28, "Swerve Drive"=w42) -> ()  [unwired: 5 in, 1 out]
    n30 = node-c288() -> ()  [unwired: 1 out]
  }
  "Align Good?" <- w2
  n31 = call "Sequence Commands.vi"("queue in"=w20) -> ()  [unwired: 11 in]
  n32 = Enqueue Element(queue=w20, element=T17 {"Time (s)"=-1.0, "Command out"={"Name"="", "vi reference"=refnum, [], []}}, error in (no error)=w19) -> ()  [unwired: 1 in, 3 out]
  n33 = node-c288(w24) -> ()
  n34 = Unbundle By Name(w9) -> ("Drive Motors (NEO)"=w14:T4, "Steer Motors (NEO)"=w13:T4)
  n35 = call "NEO Set Output.vi"("Control Mode"=w12, "Setpoints"=w11, "Motors"=w14) -> ()  [unwired: 9 in]
  n36 = call "NEO Set Output.vi"("Control Mode"=w12, "Setpoints"=w11, "Motors"=w13) -> ()  [unwired: 9 in]
